vi "LaserFinding_TwoMethods.vi"(0 "Template File Path (Pattern Matching 1)":path=path "C:/Users/reggert/Pictures/Robo/objdect.png", 7 "error in":errorcluster) -> (20 "Straight Edge (Find Vert. Edge)":T3 {"Point2 (Real-World)"."Y" format="%.2f"; "Point2 (Real-World)"."X" format="%.2f"; "Point1 (Real-World)"."Y" format="%.2f"; "Point1 (Real-World)"."X" format="%.2f"; "Point2 (Pixels)"."Y" format="%.2f"; "Point2 (Pixels)"."X" format="%.2f"; "Point1 (Pixels)"."Y" format="%.2f"; "Point1 (Pixels)"."X" format="%.2f"}, 21 "Straight Edge (Find Horiz. Edge)":T3 {"Point2 (Real-World)"."Y" format="%.2f"; "Point2 (Real-World)"."X" format="%.2f"; "Point1 (Real-World)"."Y" format="%.2f"; "Point1 (Real-World)"."X" format="%.2f"; "Point2 (Pixels)"."Y" format="%.2f"; "Point2 (Pixels)"."X" format="%.2f"; "Point1 (Pixels)"."Y" format="%.2f"; "Point1 (Pixels)"."X" format="%.2f"}, 22 "Matches (Pattern Matching 1)":T2(array[cluster]) {"Bounding Box"."y" format="%.2f"; "Bounding Box"."x" format="%.2f"; "Position"."y" format="%.2f"; "Position"."x" format="%.2f"; "Score" format="%.2f"; "Scale" format="%.2f"; "Angle" format="%.2f"}, 23 "Calibrated Matches (Pattern Matching 1)":T2(array[cluster]) {"Bounding Box"."y" format="%.2f"; "Bounding Box"."x" format="%.2f"; "Position"."y" format="%.2f"; "Position"."x" format="%.2f"; "Score" format="%.2f"; "Scale" format="%.2f"; "Angle" format="%.2f"}, 24 "Number of Matches (Pattern Matching 1)":i32, 27 "error out":errorcluster)   [LabVIEW 2014]
uses:
  <vilib>/vision/NI_Vision_Development_Module.lvlib
  <vilib>/vision/Measure.llb/Straight Edge Process.ctl
  <vilib>/vision/Measure.llb/Straight Edge Options.ctl
  <vilib>/vision/Measure.llb/Edge Polarity.ctl
  <vilib>/vision/Measure.llb/Edge Options.ctl
panel:
  out "Image Out":T1(plugin-control)
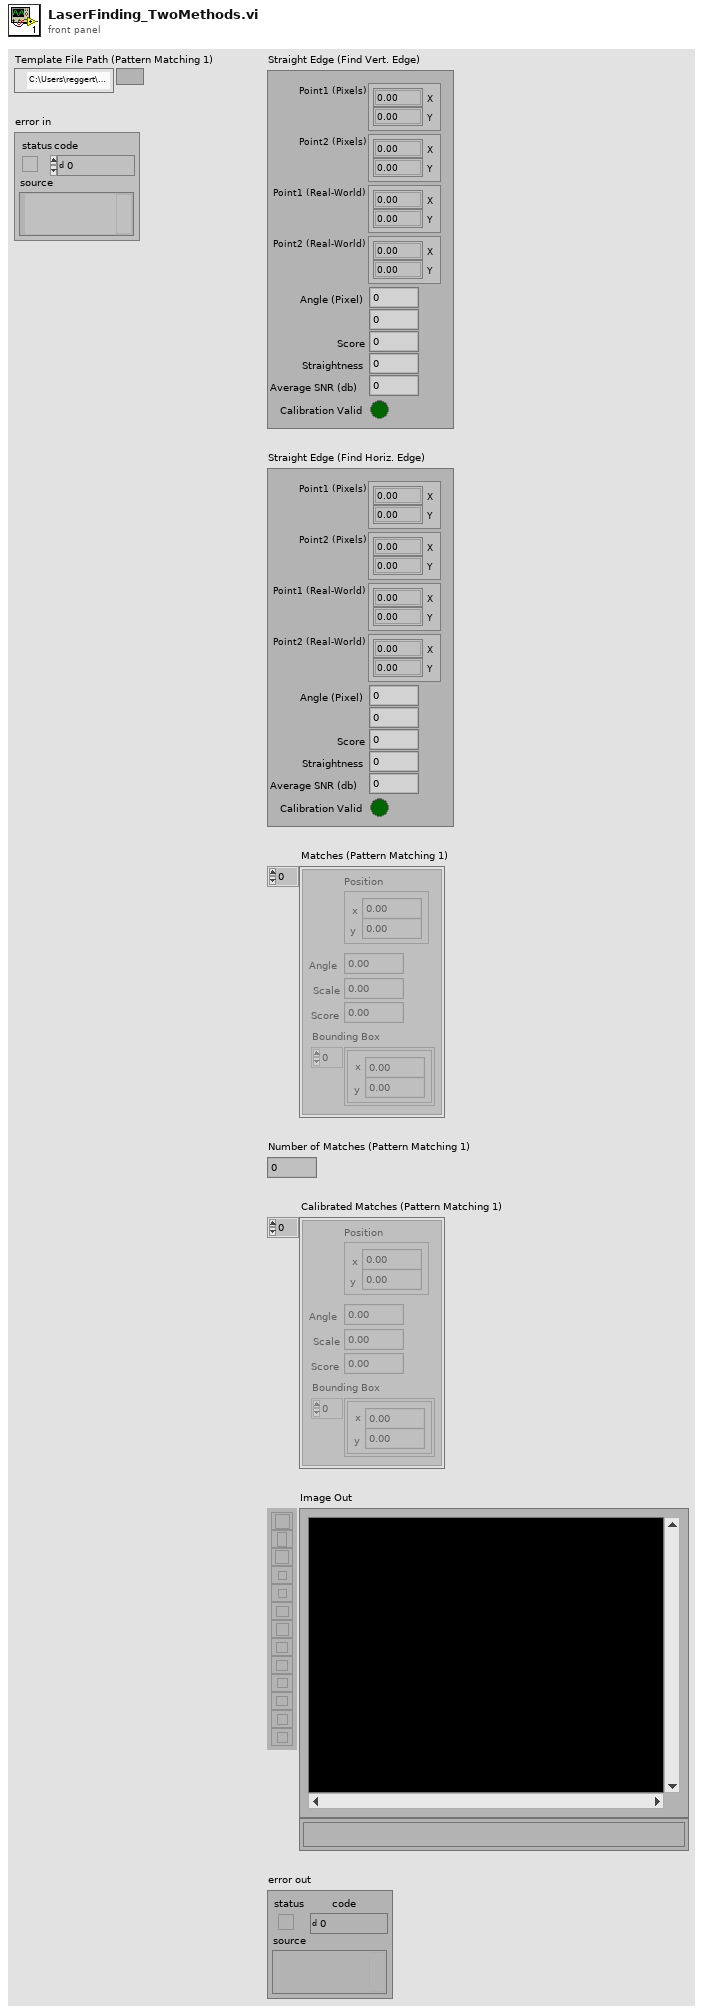
[diagram p1: front panel]
types:
  T1 = typedef "IMAQ Image.ctl" = refnum<image>
  T2 = cluster{"Position":cluster{"x":sgl, "y":sgl}, "Angle":sgl, "Scale":sgl, "Score":sgl, "Bounding Box":cluster{"x":sgl, "y":sgl}[]}[]
  T3 = cluster{"Point1 (Pixels)":cluster{"X":sgl, "Y":sgl}, "Point2 (Pixels)":cluster{"X":sgl, "Y":sgl}, "Point1 (Real-World)":cluster{"X":sgl, "Y":sgl}, "Point2 (Real-World)":cluster{"X":sgl, "Y":sgl}, "Angle (Pixel)":dbl, "Angle (Real-World)":dbl, "Score":dbl, "Straightness":dbl, "Average SNR (db)":dbl, "Calibration Valid":bool}
  T4 = cluster{"Number of Matches Requested":i32, "Minimum Match Score":sgl, "Angle Ranges":cluster{"Start Angle":sgl, "End Angle":sgl}[]}
  T5 = cluster{"Global Rectangle":i32[], "Contours":cluster{"ID":enum32{"External", "Internal"}, "Type":u32, "Coordinates":i32[]}[]}
  T6 = typedef "Edge Options.ctl" = cluster{"Edge Polarity":T7, "Kernel Size":u32, "Width":u32, "Minimum Edge Strength":sgl, "Interpolation Type":enum32{"Zero Order", "Bilinear", "Quadratic", "Cubic", "Bilinear Fixed"}, "Data Processing Method":enum32{"Average", "Median"}}
  T7 = typedef "Edge Polarity.ctl" = u32
  T8 = cluster{"Search Direction":u32, "Edge Options":T6, "Show Search Area":bool, "Show Search Lines":bool, "Show Edges Found":bool, "Show Result":bool, "Search Area Color":u32, "Search Lines Color":u32, "Edge Locations Color":u32, "Result Color":u32, "Overlay Group Name":string}
  T9 = typedef "Straight Edge Options.ctl" = cluster{"Number of Lines":i32, "Type":T10, "Min. Score":dbl, "Max. Score":dbl, "Orientation":dbl, "Angle Range":dbl, "Angle Tolerance":dbl, "Step Size":u32, "Min. SNR (db)":dbl, "Min. Points (%)":dbl, "Hough Iterations":i32}
  T10 = typedef "Straight Edge Process.ctl" = enum32{"First Edge Rake", "Best Edge Rake", "Hough Edge Rake", "First Edge Projection", "Best Edge Projection"}
  T11 = cluster{"Brightness":sgl, "Contrast":sgl, "Gamma":sgl}
  T12 = typedef "Image Type" = u32
  T13 = cluster{"Point1 (Pixels)":cluster{"X":sgl, "Y":sgl}, "Point2 (Pixels)":cluster{"X":sgl, "Y":sgl}, "Point1 (Real-World)":cluster{"X":sgl, "Y":sgl}, "Point2 (Real-World)":cluster{"X":sgl, "Y":sgl}, "Angle (Pixel)":dbl, "Angle (Real-World)":dbl, "Score":dbl, "Straightness":dbl, "Average SNR (db)":dbl, "Calibration Valid":bool}[]
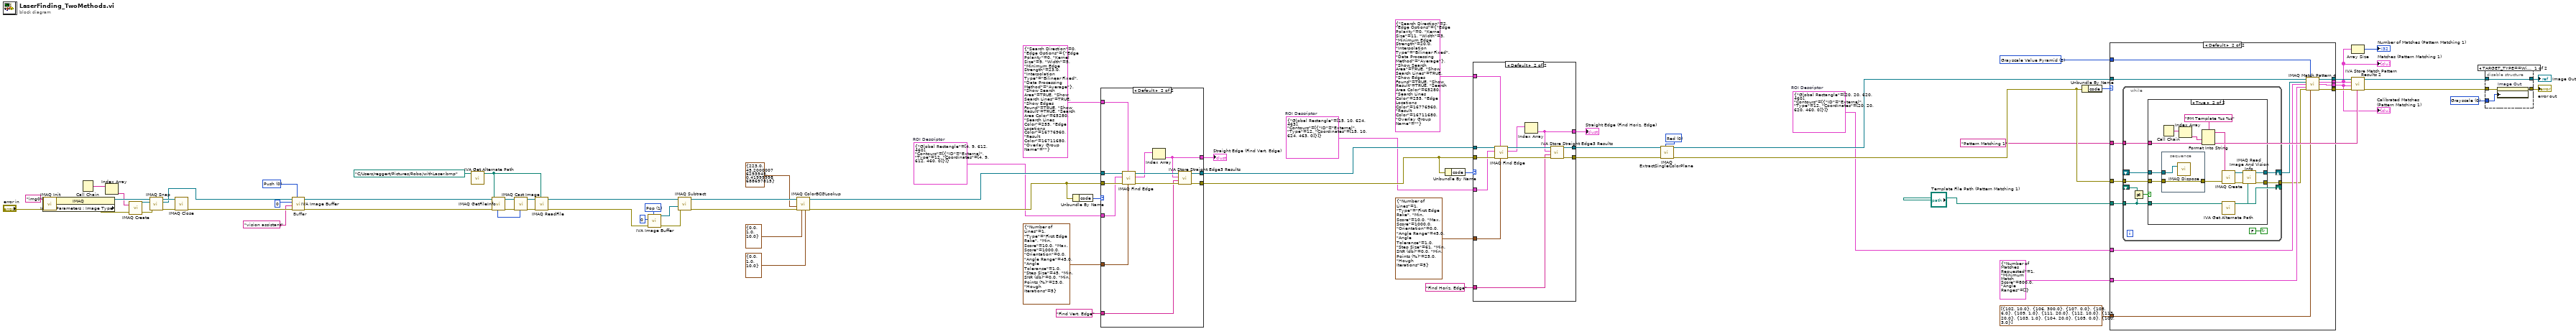
[diagram p0: block diagram]
diagram:
  w1 = u32 0 items=["Grayscale", "Binary", "Gradient", "Rainbow", "Temperature", "User Defined"] ("Palette")
  w12 = 2 items=["All", "Low Discrepancy Sampling", "Grayscale Value Pyramid", "Gradients Pyramid"] ("Algorithm")
  w7 = "Pattern Matching 1" ("Step Name")
  w11 = T5 {"Global Rectangle"=[20, 20, 620, 460], "Contours"=[{"ID"=enum."External", "Type"=12, "Coordinates"=[20, 20, 620, 460, 0]}]}  # ROI Descriptor
  w21 = 0 items=["Red", "Green", "Blue", "Hue", "Saturation", "Luminance", "Value", "Intensity"] ("Color Plane")
  w28 = T5 {"Global Rectangle"=[15, 10, 624, 463], "Contours"=[{"ID"=enum."External", "Type"=12, "Coordinates"=[15, 10, 624, 463, 0]}]}  # ROI Descriptor
  w36 = T5 {"Global Rectangle"=[4, 9, 612, 460], "Contours"=[{"ID"=enum."External", "Type"=12, "Coordinates"=[4, 9, 612, 460, 0]}]}  # ROI Descriptor
  w48 = u16 1 items=["Push", "Pop", "Reset"] ("Function")
  w59 = u16 0 items=["Push", "Pop", "Reset"] ("Function")
  # "Buffer"
  n1 = call <vilib>:"IMAQ Init.vi"("error in (no error)"="error in", "Interface Name"="img0") -> ("error out"=w68:errorcluster, "IMAQ Session Out"=w69:refnum<k11>)  [unwired: 8 out]
  n2 = property class="IMAQ" props=["Image Parameters : Image Type"](reference=w69, error in=w68) -> (reference out=w67:refnum<k11>, error out=w66:errorcluster)  [unwired: 1 out]
  n3 = Call Chain() -> (call chain=w63:string[])
  n4 = Index Array(array=w63) -> (element=w62:string)  [unwired: 1 in]
  n5 = call "IMAQ Create"("Image Name"=w62, "error in (no error)"=w66) -> ("New Image"=w73:T1, "error out"=w65:errorcluster)  [unwired: 2 in, 1 out]
  n6 = call <vilib>:"IMAQ Snap.vi"("error in (no error)"=w65, "Image In"=w73, "IMAQ Session In"=w67) -> ("error out"=w71:errorcluster, "Image Out"=w61:T1, "IMAQ Session Out"=w72:refnum<k11>)  [unwired: 6 out]
  n7 = call <vilib>:"IMAQ Close.vi"("error in (no error)"=w71, "IMAQ Session In"=w72) -> ("error out"=w70:errorcluster)  [unwired: 9 out]
  n8 = call <vilib>:"IVA Image Buffer.vi"("Function"=w59, "error in (no error)"=w70, "Prefix"="vision assistant", "Buffer #"=0, "Image In"=w61) -> ("error out"=w60:errorcluster, "Image Out"=w53:T1)  [unwired: 5 out]
  n9 = call <vilib>:"IVA Get Alternate Path.vi"("Path In"=path "C:/Users/reggert/Pictures/Robo/withLaser.bmp" ("File Path")) -> ("Path Out"=w49:path)  [unwired: 10 out]
  n10 = call "IMAQ GetFileInfo"("error in (no error)"=w60, "File Path"=w49) -> ("error out"=w55:errorcluster, "Image Type"=w51:T12)  [unwired: 8 out]
  n11 = call "IMAQ Cast Image"("Image Type"=w51, "error in (no error)"=w55, "Image Src"=w53) -> ("error out"=w54:errorcluster, "Image Dst Out"=w52:T1)  [unwired: 3 in, 4 out]
  n12 = call "IMAQ ReadFile"("File Path"=w49, "error in (no error)"=w54, "Image"=w52) -> ("error out"=w56:errorcluster, "Image Out"=w44:T1)  [unwired: 2 in, 5 out]
  n13 = call <vilib>:"IVA Image Buffer.vi"("Function"=w48, "error in (no error)"=w56, "Buffer #"=0) -> ("error out"=w45:errorcluster, "Image Out"=w46:T1)  [unwired: 2 in, 5 out]
  n14 = call "IMAQ Subtract"("Image Src A"=w44, "Image Src B"=w46, "error in (no error)"=w45) -> ("Image Dst Out"=w42:T1, "error out"=w43:errorcluster)  [unwired: 2 in, 2 out]
  n15 = call "IMAQ ColorBCGLookup"("Blue BCG Values"=T11 {"Brightness"=0.0, "Contrast"=1.0, "Gamma"=10.0}, "Green BCG Values"=T11 {"Brightness"=0.0, "Contrast"=1.0, "Gamma"=10.0}, "error in (no error)"=w43, "Red BCG Values"=T11 {"Brightness"=223.0, "Contrast"=45.2, "Gamma"=0.42}, "Image Src"=w42) -> ("error out"=w41:errorcluster, "Image Dst Out"=w37:T1)  [unwired: 2 in, 3 out]
  n16 = Unbundle By Name(w41) -> ("code"=w33:i32)
  n17 = case shown="Default" w33 {
    tunnel: w37 -> [w75 w87]
    tunnel: w41 -> [_ w86]
    tunnel: w36 -> [_ w80]
    tunnel: [w75 w84] -> w29
    tunnel: [_ w82] -> w35
    tunnel: "Find Vert. Edge" ("Step Name") -> [_ w81]
    tunnel: T9 {"Number of Lines"=1, "Type"=enum."First Edge Rake", "Min. Score"=10.0, "Max. Score"=1000.0, "Orientation"=0.0, "Angle Range"=45.0, "Angle Tolerance"=1.0, "Step Size"=45, "Min. SNR (db)"=0.0, "Min. Points (%)"=25.0, "Hough Iterations"=5} ("Fit Options") -> [_ w79]
    tunnel: T8 {"Search Direction"=0, "Edge Options"={"Edge Polarity"=0, "Kernel Size"=9, "Width"=5, "Minimum Edge Strength"=23.0, "Interpolation Type"=enum."Bilinear Fixed", "Data Processing Method"=enum."Average"}, "Show Search Area"=TRUE, "Show Search Lines"=TRUE, "Show Edges Found"=TRUE, "Show Result"=TRUE, "Search Area Color"=65280, "Search Lines Color"=255, "Edge Locations Color"=16776960, "Result Color"=16711680, "Overlay Group Name"=""} ("Options") -> [_ w78]
    tunnel: [_ w76] -> w30
    frame -1074396199, -1074396198 {
      # "Discard Coordinate System Error"
    }
    frame Default {
      n18 = call "IMAQ Find Edge"("Line Fit Options"=w79, "Options"=w78, "error in (no error)"=w86, "ROI Descriptor"=w80, "Image"=w87) -> ("error out"=w83:errorcluster, "Straight Edges"=w77:T13, "Image Out"=w85:T1)  [unwired: 1 in, 3 out]
      n19 = Index Array(array=w77) -> (element=w76:T3)  [unwired: 1 in]
      n20 = call <vilib>:"IVA Store Straight Edge3 Results.vi"("error in (no error)"=w83, "Step Name"=w81, "Straight Edge"=w76, "Image in"=w85) -> ("error out"=w82:errorcluster, "Image dup"=w84:T1)  [unwired: 1 in, 5 out]
    }
  }
  "Straight Edge (Find Vert. Edge)" <- w30
  n21 = Unbundle By Name(w35) -> ("code"=w25:i32)
  n22 = case shown="Default" w25 {
    tunnel: w29 -> [w88 w100]
    tunnel: w35 -> [_ w99]
    tunnel: w28 -> [_ w93]
    tunnel: [w88 w97] -> w20
    tunnel: [_ w95] -> w27
    tunnel: "Find Horiz. Edge" ("Step Name") -> [_ w94]
    tunnel: T9 {"Number of Lines"=1, "Type"=enum."First Edge Rake", "Min. Score"=10.0, "Max. Score"=1000.0, "Orientation"=0.0, "Angle Range"=45.0, "Angle Tolerance"=1.0, "Step Size"=61, "Min. SNR (db)"=0.0, "Min. Points (%)"=25.0, "Hough Iterations"=5} ("Fit Options") -> [_ w92]
    tunnel: T8 {"Search Direction"=2, "Edge Options"={"Edge Polarity"=0, "Kernel Size"=11, "Width"=3, "Minimum Edge Strength"=20.0, "Interpolation Type"=enum."Bilinear Fixed", "Data Processing Method"=enum."Average"}, "Show Search Area"=TRUE, "Show Search Lines"=TRUE, "Show Edges Found"=TRUE, "Show Result"=TRUE, "Search Area Color"=65280, "Search Lines Color"=255, "Edge Locations Color"=16776960, "Result Color"=16711680, "Overlay Group Name"=""} ("Options") -> [_ w91]
    tunnel: [_ w89] -> w22
    frame -1074396199, -1074396198 {
      # "Discard Coordinate System Error"
    }
    frame Default {
      n23 = call "IMAQ Find Edge"("Line Fit Options"=w92, "Options"=w91, "error in (no error)"=w99, "ROI Descriptor"=w93, "Image"=w100) -> ("error out"=w96:errorcluster, "Straight Edges"=w90:T13, "Image Out"=w98:T1)  [unwired: 1 in, 3 out]
      n24 = Index Array(array=w90) -> (element=w89:T3)  [unwired: 1 in]
      n25 = call <vilib>:"IVA Store Straight Edge3 Results.vi"("error in (no error)"=w96, "Step Name"=w94, "Straight Edge"=w89, "Image in"=w98) -> ("error out"=w95:errorcluster, "Image dup"=w97:T1)  [unwired: 1 in, 5 out]
    }
  }
  "Straight Edge (Find Horiz. Edge)" <- w22
  n26 = call "IMAQ ExtractSingleColorPlane"("Color Plane"=w21, "error in (no error)"=w27, "Image Src"=w20) -> ("error out"=w19:errorcluster, "Image Dst Out"=w17:T1)  [unwired: 1 in, 6 out]
  n27 = Unbundle By Name(w19) -> ("code"=w13:i32)
  n28 = case shown="Default" w13 {
    tunnel: "Template File Path (Pattern Matching 1)" -> [_ w115]
    tunnel: w19 -> [_ w114]
    tunnel: w17 -> [w101 w109]
    tunnel: [_ w110] -> w16
    tunnel: [_ w111] -> w6
    tunnel: [w101 w108] -> w14
    tunnel: w7 -> [_ w113]
    tunnel: w12 -> [_ w107]
    tunnel: w11 -> [_ w106]
    tunnel: T4 {"Number of Matches Requested"=1, "Minimum Match Score"=800.0, "Angle Ranges"=[]} ("Parameters") -> [_ w105]
    tunnel: cluster{"Item":u16, "Value":dbl}[] [{"Item"=102, "Value"=10.0}, {"Item"=106, "Value"=300.0}, {"Item"=107, "Value"=0.0}, {"Item"=108, "Value"=6.0}, {"Item"=109, "Value"=1.0}, {"Item"=111, "Value"=20.0}, {"Item"=112, "Value"=10.0}, {"Item"=113, "Value"=20.0}, {"Item"=103, "Value"=1.0}, {"Item"=104, "Value"=20.0}, {"Item"=105, "Value"=0.0}, {"Item"=100, "Value"=3.0}] ("Advanced Options") -> [_ w103]
    tunnel: [_ w102] -> w5
    frame -1074396199, -1074396198 {
      # "Discard Coordinate System Error"
    }
    frame Default {
      n29 = while {
        shift-right: [w124] -> w112
        shift-left: _ -> [w123]
        tunnel: [w121] -> w104
        tunnel: w114 -> [w120]
        tunnel: w115 -> [w117]
        tunnel: w113 -> [w119]
        shift-right: [w117] -> _
        shift-left: _ -> [w118]
        stop <- FALSE continue-if-true
        n30 = Not Equal?(x=w118, y=w117) -> (x != y?=w116:bool)
        n31 = case shown="True" w116 {
          tunnel: [w126 w138] -> w124
          tunnel: w123 -> [w126 w129]
          tunnel: [w125 w135] -> w121
          tunnel: w120 -> [w125 w128]
          tunnel: w117 -> [_ w131]
          tunnel: w119 -> [_ w132]
          frame False {
          }
          frame True {
            n32 = stacked-sequence {
              tunnel: w129 -> [w142]
              tunnel: w128 -> [w141]
              tunnel: [w141] -> w127
              frame #0 {
                n33 = call "IMAQ Dispose"("Image"=w142) -> ()  [unwired: 2 in, 4 out]
              }
            }
            n34 = Call Chain() -> (call chain=w134:string[])
            n35 = Index Array(array=w134) -> (element=w133:string)  [unwired: 1 in]
            n36 = Format Into String(format string="PM Template %s %s" ("Image Name"), w133, w132) -> (resulting string=w140:string)  [unwired: 2 in, 1 out]
            n37 = call "IMAQ Create"("Image Name"=w140, "error in (no error)"=w127) -> ("New Image"=w137:T1, "error out"=w136:errorcluster)  [unwired: 2 in, 1 out]
            n38 = call <vilib>:"IVA Get Alternate Path.vi"("Path In"=w131) -> ("Path Out"=w130:path)  [unwired: 10 out]
            n39 = call "IMAQ Read Image And Vision Info"("File Path"=w130, "error in (no error)"=w136, "Image"=w137) -> ("error out"=w135:errorcluster, "Image Out"=w138:T1)  [unwired: 1 in, 6 out]
          }
        }
      }
      n40 = call "IMAQ Match Pattern 4"("Image"=w109, "Algorithm"=w107, "Template Image"=w112, "ROI Descriptor"=w106, "Parameters"=w105, "error in (no error)"=w104, "Advanced Options"=w103) -> ("Image (duplicate)"=w108:T1, "Matches (pixel)"=w111:T2, "Matches (real-world)"=w102:T2, "error out"=w110:errorcluster)  [unwired: 4 in, 1 out]
    }
  }
  "Matches (Pattern Matching 1)" <- w6
  "Calibrated Matches (Pattern Matching 1)" <- w5
  n41 = Array Size(array=w6) -> (size(s)=→"Number of Matches (Pattern Matching 1)":i32)
  n42 = call <vilib>:"IVA Store Match Pattern Results 2.vi"("Step Name"=w7, "error in (no error)"=w16, "Matches (real-world)"=w5, "Matches (pixel)"=w6, "Image in"=w14) -> ("error out"=w15:errorcluster, "Image dup"=w3:T1)  [unwired: 1 in, 4 out]
  n43 = disable-structure "Conditional Disable Structure" shown="TARGET_TYPE==Windows" {
    disable-tunnel: w15 -> [w146 w147]
    disable-tunnel: [w145 w147] -> w4
    disable-tunnel: w3 -> [w144 w148]
    disable-tunnel: [w144 w148] -> w2
    disable-tunnel: w1 -> [w143 _]
    frame condition #0 (active) {
      n44 = property on="Image Out" class="ImageControl"(error in=w146, "Palette:Palette Type"=w143) -> (error out=w145:errorcluster)  [unwired: 1 in, 1 out]
    }
    frame condition #1 {
    }
  }
  "error out" <- w4
  "Image Out" <- w2
